vi "Error-Format Message.vi"(11 "error in (no error)":errorcluster) -> (4 "Message":string, 15 "No Error":errorcluster)   [LabVIEW 2020]
uses:
  Error-Library Action.ctl
  <vilib>/Utility/error.llb/DialogType.ctl
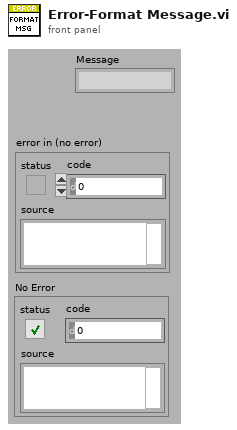
[diagram p1: front panel]
types:
  T1 = typedef "Error-Library Action.ctl" = enum16{"NONE", "Register", "Read"}
  T2 = typedef "Error Description.ctl" = cluster{"Code":i32, "Description":string, "Details":string}
  T3 = typedef "DialogType.ctl" = u16
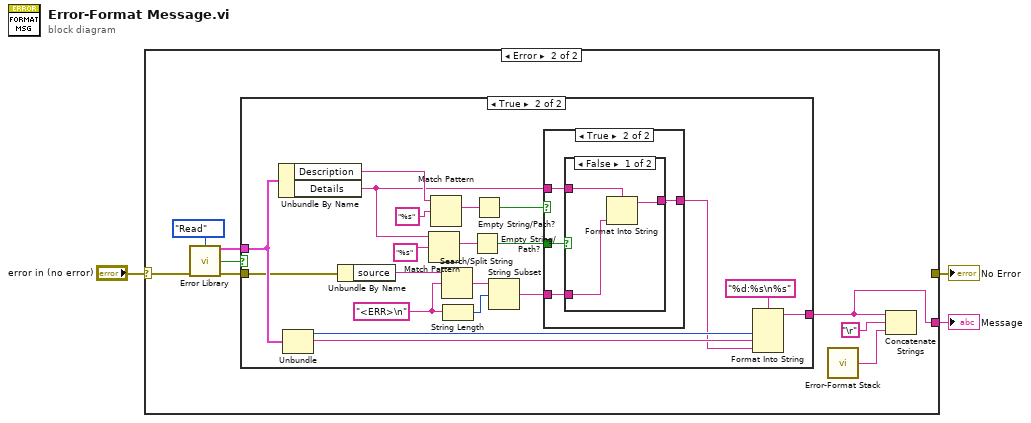
[diagram p0: block diagram]
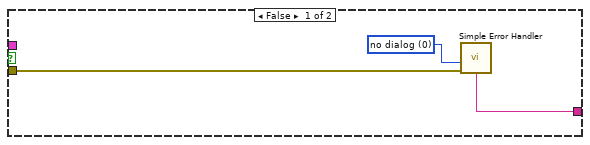
[diagram p3: hidden frame]
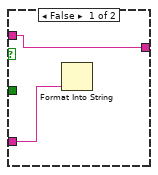
[diagram p4: hidden frame]
diagram:
  n1 = case shown="Error" "error in (no error)" {
    selector: "error in (no error)" -> [w4 w12]
    tunnel: [w4 _] -> w2
    tunnel: [_ w9] -> w1
    frame No Error {
    }
    frame Error {
      n2 = call "Error Library.vi"("action"=Error-Library_Action."Read", "error in"=w12) -> ("Entry"=w7:T2, "found?"=w5:bool, "error thru"=w6:errorcluster)  [unwired: 11 in]
      n3 = case shown="True" w5 {
        tunnel: w6 -> [w15 w17]
        tunnel: w7 -> [_ w18]
        tunnel: [w14 w33] -> w9
        frame False {
          w13 = T3 0 items=["no dialog", "OK message", "continue or stop message", "OK message + warnings", "continue/stop + warnings"] ("type of dialog (OK msg:1)")
          n4 = call <vilib>:"Simple Error Handler.vi"("type of dialog (OK msg:1)"=w13, "error in (no error)"=w15) -> ("message"=w14:string)  [unwired: 3 in, 4 out]
        }
        frame True {
          w25 = "<ERR>\n" ("search string/char (-)")
          n5 = Unbundle By Name(w18) -> ("Description"=w20:string, "Details"=w19:string)
          n6 = Unbundle(w18) -> ("Code"=w35:i32, "Description"=w34:string)  [unwired: 1 out]
          n7 = Unbundle By Name(w17) -> ("source"=w23:string)
          n8 = Match Pattern(string=w19, regular expression="%s") -> (match substring=w30:string)  [unwired: 1 in, 3 out]
          n9 = Match Pattern(string=w20, regular expression="%s") -> (match substring=w28:string)  [unwired: 1 in, 3 out]
          n10 = Search/Split String(string=w23, search string/char (-)=w25) -> (match + rest of string=w24:string)  [unwired: 1 in, 2 out]
          n11 = String Length(string=w25) -> (length=w26:i32)
          n12 = Empty String/Path?(string/path=w30) -> (empty?=w29:bool)
          n13 = Empty String/Path?(string/path=w28) -> (empty?=w22:bool)
          n14 = String Subset(string=w24, offset (0)=w26) -> (substring=w21:string)  [unwired: 1 in]
          n15 = case shown="True" w22 {
            tunnel: w29 -> [_ w41]
            tunnel: w19 -> [w37 w40]
            tunnel: [w37 w39] -> w16
            tunnel: w21 -> [w36 w38]
            frame False {
              n16 = Format Into String(w36) -> ()  [unwired: 3 in, 2 out]
            }
            frame True {
              n17 = case shown="False" w41 {
                tunnel: w40 -> [w44 w45]
                tunnel: [w43 w45] -> w39
                tunnel: w38 -> [w42 _]
                frame False {
                  n18 = Format Into String(format string=w44, w42) -> (resulting string=w43:string)  [unwired: 2 in, 1 out]
                }
                frame True {
                }
              }
            }
          }
          n19 = Format Into String(format string="%d:%s\n%s", w35, w34, w16) -> (resulting string=w33:string)  [unwired: 2 in, 1 out]
        }
      }
      n20 = call "Error-Format Stack.vi"() -> ("formatted stack"=w11:string)  [unwired: 15 in]
      n21 = Concatenate Strings(w9, "\r", w11) -> ()  [unwired: 1 out]
    }
  }
  "No Error" <- w2
  "Message" <- w1
